vi "AIT 1553 - Add Bus.vi"(7 "Called From SysDef API (F)":bool, 8 "error in (no error)":errorcluster, 10 "Bus":u16, 11 "Node Ptr":u64 format="%.0x") -> (0 "error out":errorcluster, 2 "Section Ptr Out":T1 format="%.0x")   [LabVIEW 2013, in "AIT 1553 Custom Device.lvlib"]
uses:
  AIT 1553 Custom Device.lvlib
  <vilib>/NI Veristand/Custom Device API/Custom Device Item Ref.ctl
  Controls and Global/Global.vi
  <vilib>/NI Veristand/Custom Device API/Set Item Property (U16).vi
  <vilib>/NI Veristand/Custom Device API/Custom Device API.lvlib
  <vilib>/NI Veristand/Custom Device Tools/Custom Device Utility Library/Custom Device Utility Library.lvlib
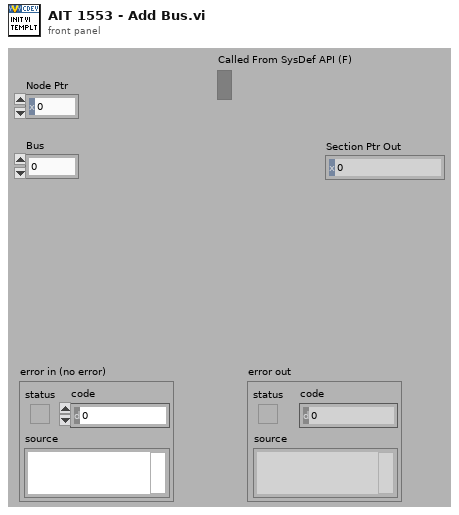
[diagram p1: front panel]
types:
  T1 = typedef "Custom Device API.lvlib/Custom Device Item Ref.ctl" = u64
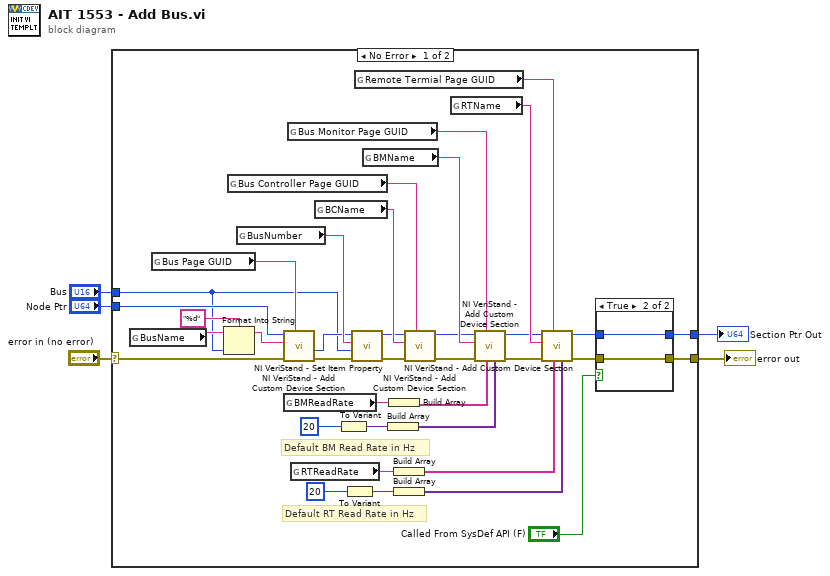
[diagram p0: block diagram]
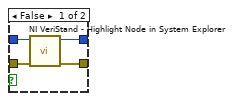
[diagram p2: hidden frame]
diagram:
  n1 = case shown="No Error" "error in (no error)" {
    selector: "error in (no error)" -> [w41 w49]
    tunnel: "Node Ptr" -> [w42 _]
    tunnel: [w40 w49] -> w3
    tunnel: "Bus" -> [w18 _]
    tunnel: [w11 _] -> w1
    frame No Error {
      # "Default RT Read Rate in Hz"
      # "Default BM Read Rate in Hz"
      n2 = global read "Global.vi" "BusName"() -> (w19:string)
      n3 = global read "Global.vi" "Bus Page GUID"() -> (w21:string)
      n4 = Format Into String(format string="%d", initial string=w19, w18) -> (resulting string=w32:string)  [unwired: 1 in, 1 out]
      n5 = global read "Global.vi" "Bus Controller Page GUID"() -> (w24:string)
      n6 = global read "Global.vi" "BusNumber"() -> (w34:string)
      n7 = call <vilib>:"NI VeriStand - Add Custom Device Section.vi"("GUID (Default Section)"=w21, "error in (no error)"=w41, "Section Name"=w32, "Parent Ref in"=w42) -> ("error out"=w35:errorcluster, "Section Ptr"=w33:T1)  [unwired: 4 in, 2 out]
      n8 = global read "Global.vi" "BMReadRate"() -> (w17:string)
      n9 = global read "Global.vi" "Bus Monitor Page GUID"() -> (w23:string)
      n10 = global read "Global.vi" "RTReadRate"() -> (w10:string)
      n11 = global read "Global.vi" "BCName"() -> (w39:string)
      n12 = To Variant(anything=u16 20) -> (Variant=w15:variant)
      n13 = To Variant(anything=u16 20) -> (Variant=w7:variant)
      n14 = call-poly <vilib>:"NI VeriStand - Set Item Property.vi"("error in (no error)"=w35, "Value"=w18, "Property Name"=w34, "Item Ref in"=w33) -> ("error out"=w36:errorcluster, "Item Ref out"=w27:T1)  [unwired: 5 in, 1 out]
      n15 = global read "Global.vi" "Remote Termial Page GUID"() -> (w22:string)
      n16 = global read "Global.vi" "BMName"() -> (w38:string)
      n17 = Build Array(w15) -> (w13:variant[])
      n18 = Build Array(w17) -> (w16:string[])
      n19 = Build Array(w10) -> (w9:string[])
      n20 = Build Array(w7) -> (w6:variant[])
      n21 = call <vilib>:"NI VeriStand - Add Custom Device Section.vi"("GUID (Default Section)"=w24, "error in (no error)"=w36, "Section Name"=w39, "Parent Ref in"=w27) -> ("error out"=w30:errorcluster, "Parent Ref out"=w31:T1)  [unwired: 4 in, 2 out]
      n22 = global read "Global.vi" "RTName"() -> (w37:string)
      n23 = call <vilib>:"NI VeriStand - Add Custom Device Section.vi"("Property Values"=w13, "Property names"=w16, "GUID (Default Section)"=w23, "error in (no error)"=w30, "Section Name"=w38, "Parent Ref in"=w31) -> ("error out"=w29:errorcluster, "Parent Ref out"=w28:T1)  [unwired: 2 in, 2 out]
      n24 = call <vilib>:"NI VeriStand - Add Custom Device Section.vi"("Property Values"=w6, "Property names"=w9, "GUID (Default Section)"=w22, "error in (no error)"=w29, "Section Name"=w37, "Parent Ref in"=w28) -> ("error out"=w26:errorcluster, "Parent Ref out"=w25:T1)  [unwired: 2 in, 2 out]
      n25 = case shown="True" "Called From SysDef API (F)" {
        tunnel: [w46 w48] -> w40
        tunnel: w26 -> [w45 w48]
        tunnel: w25 -> [w44 w47]
        tunnel: [w43 w47] -> w11
        frame False {
          n26 = call <vilib>:"NI VeriStand - Highlight Node in System Explorer.vi"("error in (no error)"=w45, "Item Ref in"=w44) -> ("error out"=w46:errorcluster, "Node Ptr dup"=w43:T1)  [unwired: 8 in]
        }
        frame True {
        }
      }
    }
    frame Error {
    }
  }
  "error out" <- w3
  "Section Ptr Out" <- w1
